vi "Barcode-Indentify-Close_Api.vi"(8 "Error In":errorcluster, 11 "Progressing Data":T3) -> (0 "Error Out":errorcluster)   [LabVIEW 2019]
uses:
  <vilib>/vision/Image Controls.llb/IMAQ Image.ctl
  <vilib>/userDefined/High Color/IMAQdx.ctl
  <vilib>/vision/driver/NI_Vision_Acquisition_Software.lvlib
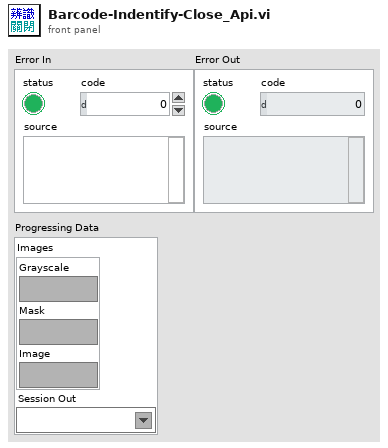
[diagram p1: front panel]
types:
  T1 = typedef "IMAQ Image.ctl" = refnum<image>
  T2 = typedef "IMAQdx.ctl" = refnum<k21>
  T3 = cluster{"Images":cluster{"Grayscale":T1, "Mask":T1, "Image":T1}, "Session Out":T2}
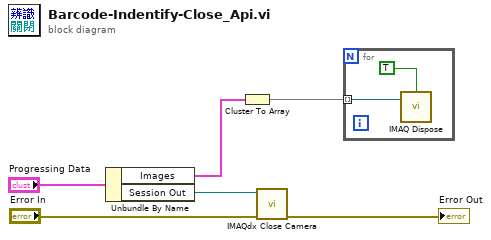
[diagram p0: block diagram]
diagram:
  n1 = Unbundle By Name("Progressing Data") -> ("Images"=w3:cluster{"Grayscale":T1, "Mask":T1, "Image":T1}, "Session Out"=w2:T2)
  n2 = Cluster To Array(cluster=w3) -> (array=w5:T1[])
  n3 = call <vilib>:"IMAQdx Close Camera.vi"("error in"="Error In", "Session In"=w2) -> ("error out"=→"Error Out":errorcluster)  [unwired: 9 in]
  n4 = for {
    tunnel: w5 -> [w8] mode=indexing
    n5 = call "IMAQ Dispose"("All Images? (No)"=TRUE, "Image"=w8) -> ()  [unwired: 4 in, 1 out]
  }
